vi "Gray's Mod Motor Controler Test Compile.vi"() -> ()   [LabVIEW 2009]
uses:
  Motor Control/Motor Control Global.vi
  Motor Control/Inner Control/Drive Control Global.vi
  Motor Control/Motor Output Global.vi
panel:
  out "Steering Output Command":fxp<+/-,20,5>
  out "Steering Output Voltage":fxp<+/-,20,5>
  in  "Steering Enable":bool
  in  "Lidar Output Voltage":fxp<+/-,20,5>
  in  "Lidar Output Command":fxp<+/-,20,5>
  in  "Lidar Enable":bool
  out "Drive Reverse":bool
  out "Drive Output Voltage":fxp<+/-,20,5>
  out "Drive Output Command":fxp<+/-,20,5>
  in  "Drive Enable":bool
  in  "Directly Output Drive Setpoint as Voltage":bool
  out "Drive Encoder tick/count":u32
  out "# of ticks/count recorded":i32
  out "Drive Encoder ft/sec 2":fxp<+/-,18,8>
  in  "Lidar Encoder Cap":i32
  out "Lidar Encoder Sub Index":i32
  out "Lidar Phi_B":fxp<+/-,14,4>
  out "Lidar Phi_A":fxp<+/-,14,4>
  out "Lidar Speed, Measured (ft/sec)":fxp<+/-,14,4>
  in  "Lidar Speed Control Integral Feedback Gain":fxp<+/-,20,5>
  in  "Lidar Speed Control Feedback Gain":fxp<+/-,20,5>
  in  "Lidar Phi_B Set Point (pi rad)":fxp<+/-,14,4>
  out "Lidar Encoder Delta":i32
  in  "stop":bool
  in  "Steering Integral Control Feedback Gain":fxp<+/-,20,5>
  in  "Steering Position Offset":i32
  in  "Steering Position Set Point (degrees)":i32
  in  "Steering Proportional Control Feedback Gain":fxp<+/-,20,5>
  out "Drive Speed, Measured (ft/sec)":fxp<+/-,14,4>
  in  "Drive Speed Control Integral Feedback Gain":fxp<+/-,20,-3>
  in  "Drive Speed Control Feedback Gain":fxp<+/-,20,5>
  in  "Drive Speed Set Point (ft/sec)":fxp<+/-,14,4>
  in  "Drive Encoder Delta":i32
  # "Drive Motor Control"
  # "Steering Motor Control"
  # "Lidar Motor Control"
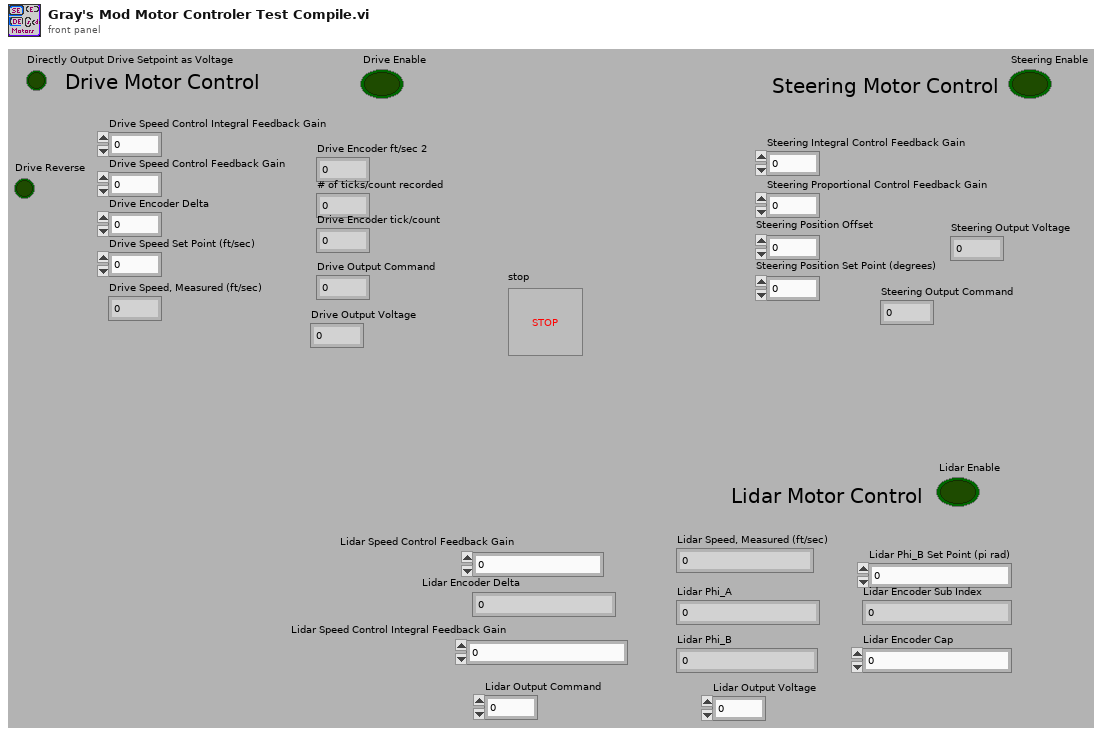
[diagram p1: front panel]
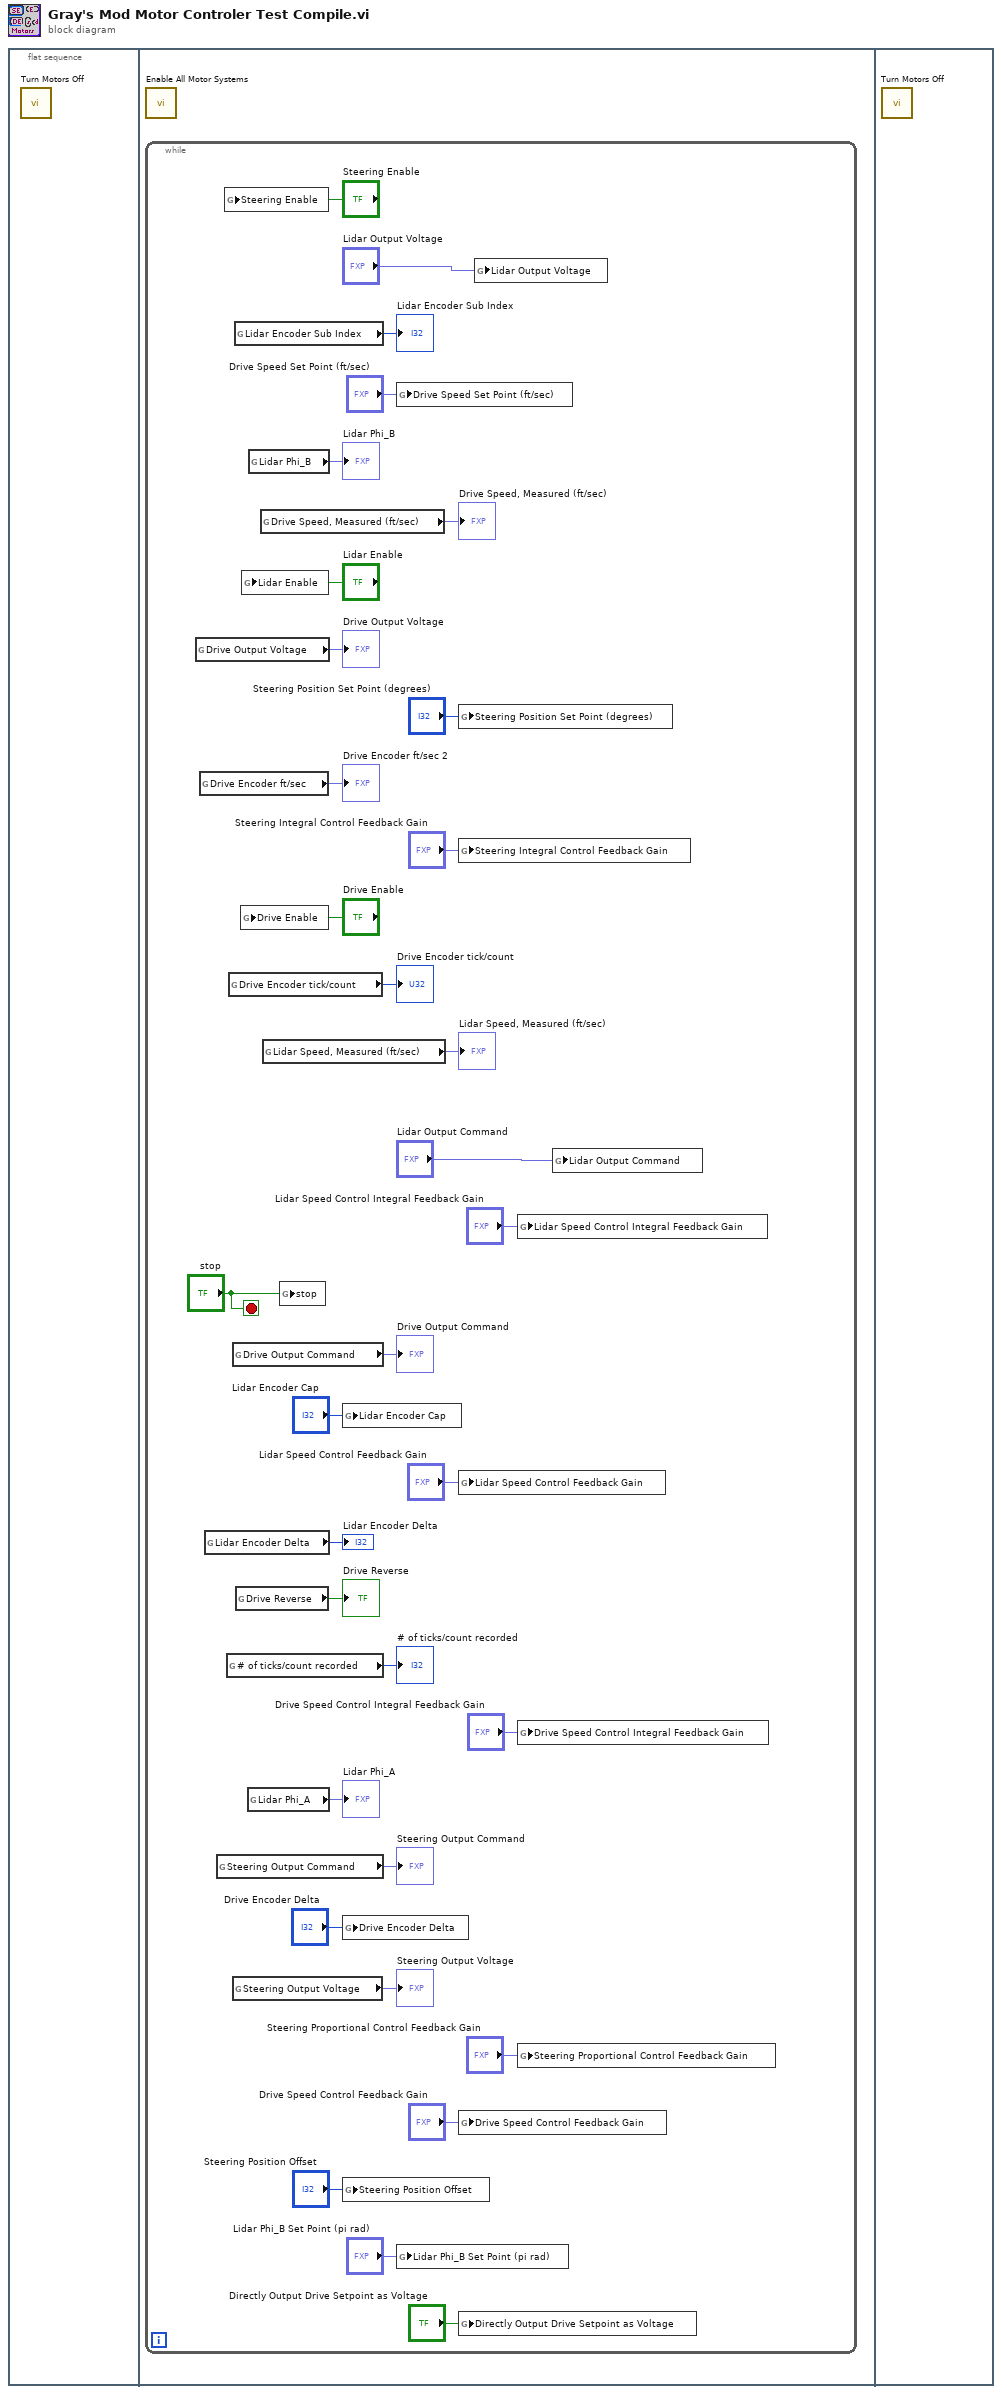
[diagram p0: block diagram]
diagram:
  n1 = flat-sequence {
    frame #0 {
      n2 = call "Turn Motors Off.vi"() -> ()  [unwired: 1 in]
    }
    frame #1 {
      n3 = call "Enable All Motor Systems.vi"() -> ()  [unwired: 1 in]
      n4 = while {
        stop <- "stop" stop-if-true
        n5 = global read "Motor Output Global.vi" "Drive Output Voltage"() -> (→"Drive Output Voltage":fxp<+/-,20,5>)
        n6 = global read "Drive Control Global.vi" "Drive Encoder ft/sec"() -> (→"Drive Encoder ft/sec 2":fxp<+/-,18,8>)
        n7 = global read "Motor Control Global.vi" "Lidar Encoder Delta"() -> (→"Lidar Encoder Delta":i32)
        n8 = global read "Motor Output Global.vi" "Steering Output Command"() -> (→"Steering Output Command":fxp<+/-,20,5>)
        n9 = global write "Motor Output Global.vi" "Steering Enable"("Steering Enable") -> ()
        n10 = global read "Drive Control Global.vi" "# of ticks/count recorded"() -> (→"# of ticks/count recorded":i32)
        n11 = global read "Drive Control Global.vi" "Drive Encoder tick/count"() -> (→"Drive Encoder tick/count":u32)
        n12 = global read "Motor Output Global.vi" "Drive Output Command"() -> (→"Drive Output Command":fxp<+/-,20,5>)
        n13 = global read "Motor Output Global.vi" "Steering Output Voltage"() -> (→"Steering Output Voltage":fxp<+/-,20,5>)
        n14 = global read "Motor Control Global.vi" "Lidar Encoder Sub Index"() -> (→"Lidar Encoder Sub Index":i32)
        n15 = global read "Motor Output Global.vi" "Drive Reverse"() -> (→"Drive Reverse":bool)
        n16 = global write "Motor Output Global.vi" "Drive Enable"("Drive Enable") -> ()
        n17 = global write "Motor Output Global.vi" "Lidar Enable"("Lidar Enable") -> ()
        n18 = global read "Motor Control Global.vi" "Lidar Phi_A"() -> (→"Lidar Phi_A":fxp<+/-,10,1>)
        n19 = global read "Motor Control Global.vi" "Lidar Phi_B"() -> (→"Lidar Phi_B":fxp<+/-,10,1>)
        n20 = global read "Motor Control Global.vi" "Drive Speed, Measured (ft/sec)"() -> (→"Drive Speed, Measured (ft/sec)":fxp<+/-,14,4>)
        n21 = global read "Motor Control Global.vi" "Lidar Speed, Measured (ft/sec)"() -> (→"Lidar Speed, Measured (ft/sec)":fxp<+/-,14,4>)
        n22 = global write "Motor Control Global.vi" "stop"("stop") -> ()
        n23 = global write "Motor Control Global.vi" "Lidar Encoder Cap"("Lidar Encoder Cap") -> ()
        n24 = global write "Motor Control Global.vi" "Drive Encoder Delta"("Drive Encoder Delta") -> ()
        n25 = global write "Motor Control Global.vi" "Steering Position Offset"("Steering Position Offset") -> ()
        n26 = global write "Motor Control Global.vi" "Drive Speed Set Point (ft/sec)"("Drive Speed Set Point (ft/sec)") -> ()
        n27 = global write "Motor Control Global.vi" "Lidar Phi_B Set Point (pi rad)"("Lidar Phi_B Set Point (pi rad)") -> ()
        n28 = global write "Motor Control Global.vi" "Steering Position Set Point (degrees)"("Steering Position Set Point (degrees)") -> ()
        n29 = global write "Motor Control Global.vi" "Steering Integral Control Feedback Gain"("Steering Integral Control Feedback Gain") -> ()
        n30 = global write "Motor Control Global.vi" "Lidar Speed Control Feedback Gain"("Lidar Speed Control Feedback Gain") -> ()
        n31 = global write "Motor Control Global.vi" "Drive Speed Control Feedback Gain"("Drive Speed Control Feedback Gain") -> ()
        n32 = global write "Motor Control Global.vi" "Directly Output Drive Setpoint as Voltage"("Directly Output Drive Setpoint as Voltage") -> ()
        n33 = global write "Motor Output Global.vi" "Lidar Output Voltage"("Lidar Output Voltage") -> ()
        n34 = global write "Motor Control Global.vi" "Lidar Speed Control Integral Feedback Gain"("Lidar Speed Control Integral Feedback Gain") -> ()
        n35 = global write "Motor Control Global.vi" "Drive Speed Control Integral Feedback Gain"("Drive Speed Control Integral Feedback Gain") -> ()
        n36 = global write "Motor Control Global.vi" "Steering Proportional Control Feedback Gain"("Steering Proportional Control Feedback Gain") -> ()
        n37 = global write "Motor Output Global.vi" "Lidar Output Command"("Lidar Output Command") -> ()
      }
    }
    frame #2 {
      n38 = call "Turn Motors Off.vi"() -> ()  [unwired: 1 in]
    }
  }
